vi "IF2_EventRead.vi"(8 "error in (no error)":errorcluster, 11 "TCP Network Connection in":refnum<k5>) -> (0 "error out":errorcluster, 2 "data out":string, 3 "TCP Network Connection out":refnum<k5>, 4 "Timeout":bool)   [LabVIEW 2015, in "IF2_Reader.lvlib"]
uses:
  IF2_Reader.lvlib
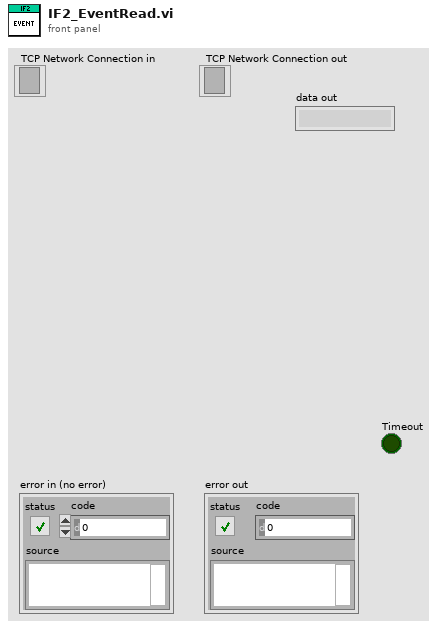
[diagram p1: front panel]
types:
  T1 = enum16{"Standard", "Buffered", "CRLF", "Immediate"}
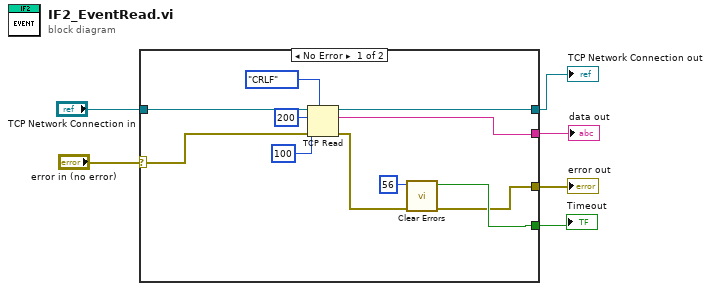
[diagram p0: block diagram]
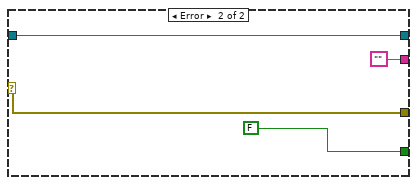
[diagram p2: hidden frame]
diagram:
  n1 = case shown="No Error" "error in (no error)" {
    selector: "error in (no error)" -> [w15 w20]
    tunnel: "TCP Network Connection in" -> [w16 w21]
    tunnel: [w17 w21] -> w4
    tunnel: [w12 w20] -> w6
    tunnel: [w13 FALSE] -> w2
    tunnel: [w7 ""] -> w1
    frame No Error {
      n2 = TCP Read(connection ID=w16, bytes to read=200, error in (no error)=w15, 7:T1."CRLF" ("mode (standard)"), 9:100 ("timeout ms (25000)")) -> (connection ID out=w17:refnum<k5>, data out=w7:string, error out=w11:errorcluster)
      n3 = call <vilib>:"Clear Errors.vi"("error in (no error)"=w11, "specific error code to clear (0: all)"=56) -> ("error out"=w12:errorcluster, "specific error cleared?"=w13:bool)  [unwired: 4 in]
    }
    frame Error {
    }
  }
  "TCP Network Connection out" <- w4
  "error out" <- w6
  "Timeout" <- w2
  "data out" <- w1
